vi "get_result_from_queue.vi"(8 "error in (no error)":errorcluster, 11 "Plots in":refnum<class "Plots.lvclass">) -> (0 "error out":errorcluster, 2 "result":string, 3 "Plots out":refnum<class "Plots.lvclass">)   [LabVIEW 2017, in "Plots.lvclass"]
doc: "reads the string from the results queue and therefor removes it out of the queue"
uses:
  Plots.lvclass
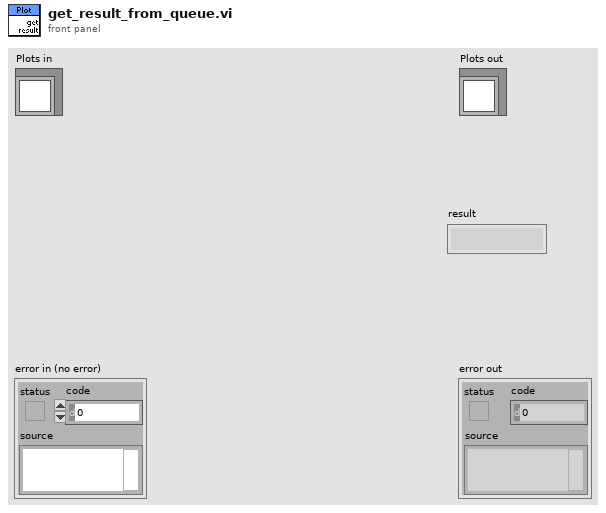
[diagram p1: front panel]
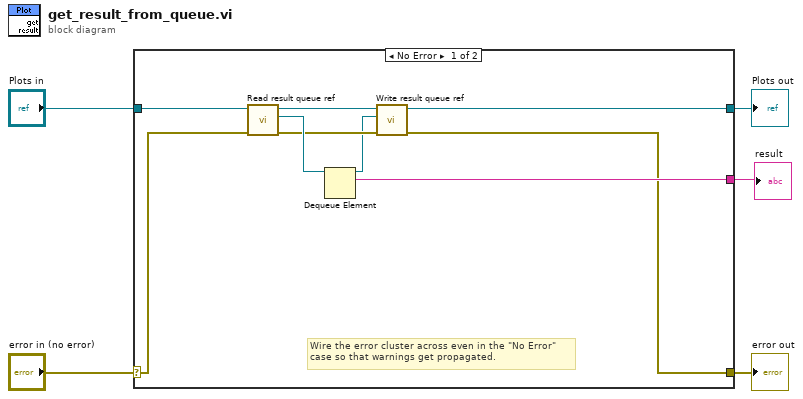
[diagram p0: block diagram]
diagram:
  n1 = case shown="No Error" "error in (no error)" {
    selector: "error in (no error)" -> [w8 w16]
    tunnel: [w7 w16] -> w4
    tunnel: [w9 w15] -> w2
    tunnel: "Plots in" -> [w14 w15]
    tunnel: [w12 _] -> w1
    frame No Error {
      # "Wire the error cluster across even in the \"No Error\"\ncase so that warnings get propagated."
      n2 = call-dynamic "Read result queue ref.vi"("error in (no error)"=w8, "Plots in"=w14) -> ("error out"=w10:errorcluster, "result queue ref"=w13:refnum<queue>, "Plots out"=w11:refnum<class "Plots.lvclass">)  [unwired: 7 in]
      n3 = Dequeue Element(queue=w13) -> (queue out=w6:refnum<queue>, element=w12:string)  [unwired: 2 in, 2 out]
      n4 = call-dynamic "Write result queue ref.vi"("error in (no error)"=w10, "result queue ref"=w6, "Plots in"=w11) -> ("error out"=w7:errorcluster, "Plots out"=w9:refnum<class "Plots.lvclass">)  [unwired: 7 in]
    }
    frame Error {
    }
  }
  "error out" <- w4
  "Plots out" <- w2
  "result" <- w1
